vi "MongoDB.FindOneByID.vi"(8 "error in (no error)":errorcluster, 10 "JSON Query String":string, 11 "MongoDB.Collection in":refnum<class "MongoDB.Collection.lvclass">) -> (0 "error out":errorcluster, 2 "Result":string, 3 "MongoDB.Collection out":refnum<class "MongoDB.Collection.lvclass">)   [LabVIEW 2014, in "MongoDB.Collection.lvclass"]
uses:
  MongoDB.Collection.lvclass
  C:/Users/Richard/Documents/GitHub/mongo-labview-driver/CSharp/bin/MongoDB.Bson.dll
  CSharp/bin/MongoDB.Bson.dll
  MongoDB.Collection.lvclass/MongoDB.Collection.ctl
  C:/Users/Richard/Documents/GitHub/mongo-labview-driver/CSharp/bin/MongoDB.Driver.Legacy.dll
  CSharp/bin/MongoDB.Driver.Legacy.dll
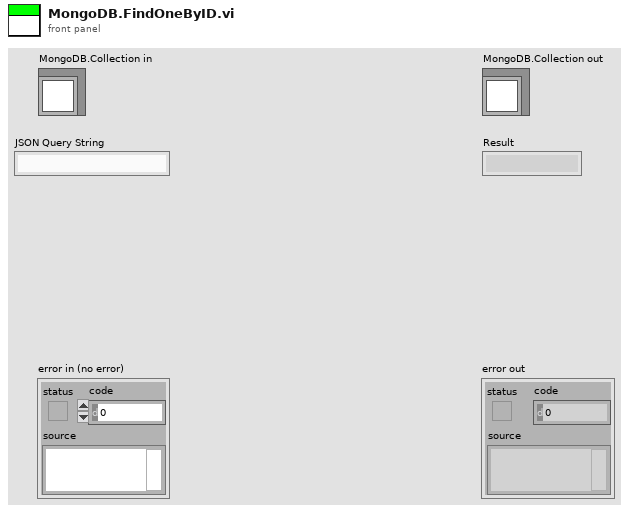
[diagram p1: front panel]
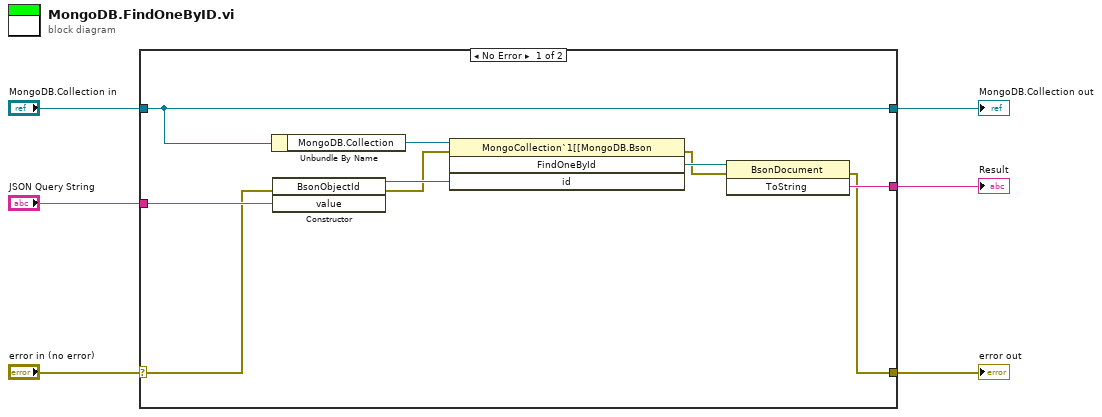
[diagram p0: block diagram]
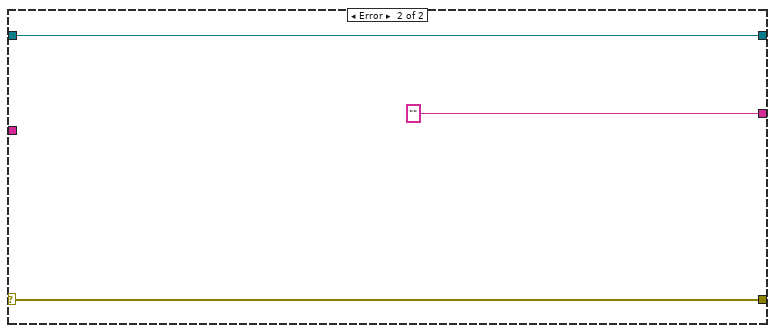
[diagram p2: hidden frame]
diagram:
  n1 = case shown="No Error" "error in (no error)" {
    selector: "error in (no error)" -> [w8 w19]
    tunnel: [w11 w19] -> w5
    tunnel: [w16 w18] -> w3
    tunnel: "MongoDB.Collection in" -> [w16 w18]
    tunnel: "JSON Query String" -> [w10 _]
    tunnel: [w13 "" ("ToString")] -> w1
    frame No Error {
      n2 = Unbundle By Name(w16) -> ("MongoDB.Collection"=w15:refnum<k24>)
      n3 = constructor class="BsonObjectId"(error in=w8, "value"=w10) -> (reference out=w9:refnum<k24>, error out=w7:errorcluster)  [unwired: 2 in, 2 out]
      n4 = invoke class="MongoCollection`1[[MongoDB.Bson" method="FindOneById"(reference=w15, error in=w7, "id"=w9) -> (error out=w12:errorcluster, "FindOneById"=w14:refnum<k24>)  [unwired: 1 in, 2 out]
      n5 = invoke class="BsonDocument" method="ToString"(reference=w14, error in=w12) -> (error out=w11:errorcluster, "ToString"=w13:string)  [unwired: 1 in, 1 out]
    }
    frame Error {
    }
  }
  "error out" <- w5
  "MongoDB.Collection out" <- w3
  "Result" <- w1
